vi "DebugMachine Viewer.vi"() -> ()   [LabVIEW 2009]
uses:
  Debug Data Packet.ctl
  TypeDefs/State Machine/Main State.ctl
  cRIO/Functional Global Variables/Status Indicators.ctl
  TypeDefs/Sensor TypeDefs/GPS Data.ctl
  TypeDefs/Sensor TypeDefs/SICK Array.ctl
  Remote Control/Motor Command.ctl
  TypeDefs/Queue TypeDefs/Motor Instruction.ctl
  TypeDefs/Queue TypeDefs/Motor State.ctl
  UDP Lib/UDP Network Location.ctl
  <vilib>/Platform/TimedLoop/XDataNode/XDataNode.xnode
  <vilib>/Platform/TimedLoop/XDataNode/loadlvalarms.vi
  <vilib>/Platform/TimedLoop/XDataNode/timing_clust.ctl
  <vilib>/Platform/TimedLoop/XDataNode/nitl_modes.ctl
  <vilib>/Platform/TimedLoop/XDataNode/wakeup.ctl
  <vilib>/Platform/TimedLoop/XDataNode/XDNodeRunTimeDep.lvlib
panel:
  out "Corrupt Data":bool=TRUE
  in  "Compact RIO Location":T1={"IP Address"="192.168.1.2", "Port"=50004}
  out "Viewer Start time":timestamp=timestamp(3355340375.117 s since 1904-01-01)
  out "Time of most recent data":timestamp=timestamp(3355340545.74 s since 1904-01-01)
  out "Iteration Duration":i64=1000
  out "Timeout":bool=TRUE
  out "HB":bool=TRUE
  in  "stop":bool
  out "Sender Network Location":T1={"IP Address"="0.0.0.0", "Port"=0}
  out "Cluster":T2={"Main State out"=enum."Initialize Sensors", "HB out"=FALSE, "Status Indicators out"={"GPS Init Complete"=FALSE, "SICK Init Complete"=FALSE, "Compass Init Complete"=FALSE, "Camera Init Complete"=FALSE, "Sensors Init Complete"=FALSE, "Motors Init Complete"=FALSE, "MC Heartbeat"=FALSE, "Motors On?"=FALSE}, "RC/!Run out"=TRUE, "AUT/!NAV"=FALSE, "Compass Data"=0.0, "GPS Data"={"Latitude"=0.0, "Longitude"=0.0}, "SICK Data"=[], "Target Bearing"=0.0, "Target Sector"=0, "Calculated sector"=0, "RC Command"={"Speed"=0, "Turn"=0}, "Motor Loop Instruction"={"Motor State"=enum."Stop", "Motor Command"={"Speed"=0, "Turn"=0}}, "Waypoints reached"=0, "Battery Voltage"=0.0} {"GPS Data"."Longitude" format="%#_14g"; "GPS Data"."Latitude" format="%#_14g"}
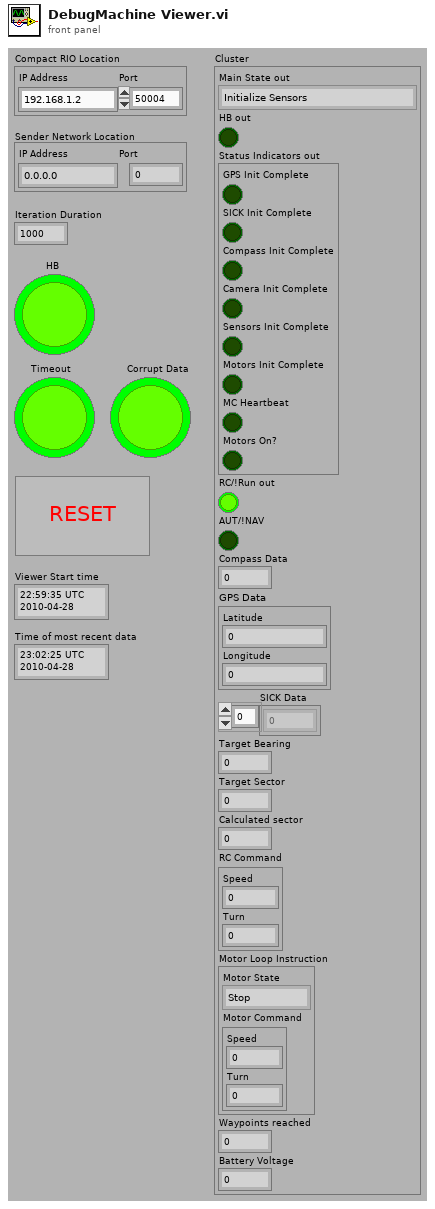
[diagram p1: front panel]
types:
  T1 = typedef "UDP Network Location.ctl" = cluster{"IP Address":string, "Port":u16}
  T2 = typedef "Debug Data Packet.ctl" = cluster{"Main State out":T3, "HB out":bool, "Status Indicators out":T4, "RC/!Run out":bool, "AUT/!NAV":bool, "Compass Data":dbl, "GPS Data":T5, "SICK Data":T6, "Target Bearing":dbl, "Target Sector":i16, "Calculated sector":i16, "RC Command":T7, "Motor Loop Instruction":T8, "Waypoints reached":i8, "Battery Voltage":dbl}
  T3 = typedef "Main State.ctl" = enum16{"Initialize Sensors", "Initialize Motors", "Wait for GO", "Run", "Remote Control", "Stop"}
  T4 = typedef "Status Indicators.ctl" = cluster{"GPS Init Complete":bool, "SICK Init Complete":bool, "Compass Init Complete":bool, "Camera Init Complete":bool, "Sensors Init Complete":bool, "Motors Init Complete":bool, "MC Heartbeat":bool, "Motors On?":bool}
  T5 = typedef "GPS Data.ctl" = cluster{"Latitude":dbl, "Longitude":dbl}
  T6 = typedef "SICK Array.ctl" = u16[]
  T7 = typedef "Motor Command.ctl" = cluster{"Speed":i16, "Turn":i16}
  T8 = typedef "Motor Instruction.ctl" = cluster{"Motor State":T9, "Motor Command":T7}
  T9 = typedef "Motor State.ctl" = enum16{"Wait", "Initialize", "Check FET", "Run", "Stop"}
  T10 = typedef "XDNodeRunTimeDep.lvlib/timing_clust.ctl" = cluster{"Expected End [f-1]":u64, "Actual End [f-1]":u64, "Finished Late? [f-1]":bool, "Expected End [i-1]":u64, "Actual End [i-1]":u64, "Finished Late? [i-1]":bool, "Expected Start [i]":u64, "Actual Start [i]":u64, "Expected Start [f]":u64, "Actual Start [f]":u64, "Source Name":string, "Structure Name":string, "Period":i64, "Deadline":i64, "Offset":i64, "Start":i64, "Priority":i32, "Timeout":i32, "Mode":T11, "Wakeup Reason":T12, "Error":errorcluster, "Source Type":string, "Secondary Source Type":string, "Global End Time":u64, "Global Start Time":u64, "Frame Duration":u64, "Iteration Duration":u64, "Assigned CPU":i32, "I/O Scan Engine Mode":u32}
  T11 = typedef "XDNodeRunTimeDep.lvlib/nitl_modes.ctl" = enum32{"No Change", "Process missed periods, maintain original phase", "Discard missed periods, maintain original phase", "Process missed periods, ignore original phase", "Discard missed periods, ignore original phase"}
  T12 = typedef "XDNodeRunTimeDep.lvlib/wakeup.ctl" = enum32{"Normal", "Aborted", "Asynchronous wakeup", "Timing source error", "Timed loop error", "Timeout"}
  T13 = typedef "UDP Base.ctl" = cluster{"UDP Session":refnum<k16>, "UDP Socket Params":T14}
  T14 = typedef "UDP Socket Params.ctl" = cluster{"Local Port":u16, "Read Timeout":i32, "Write Timeout":i32}
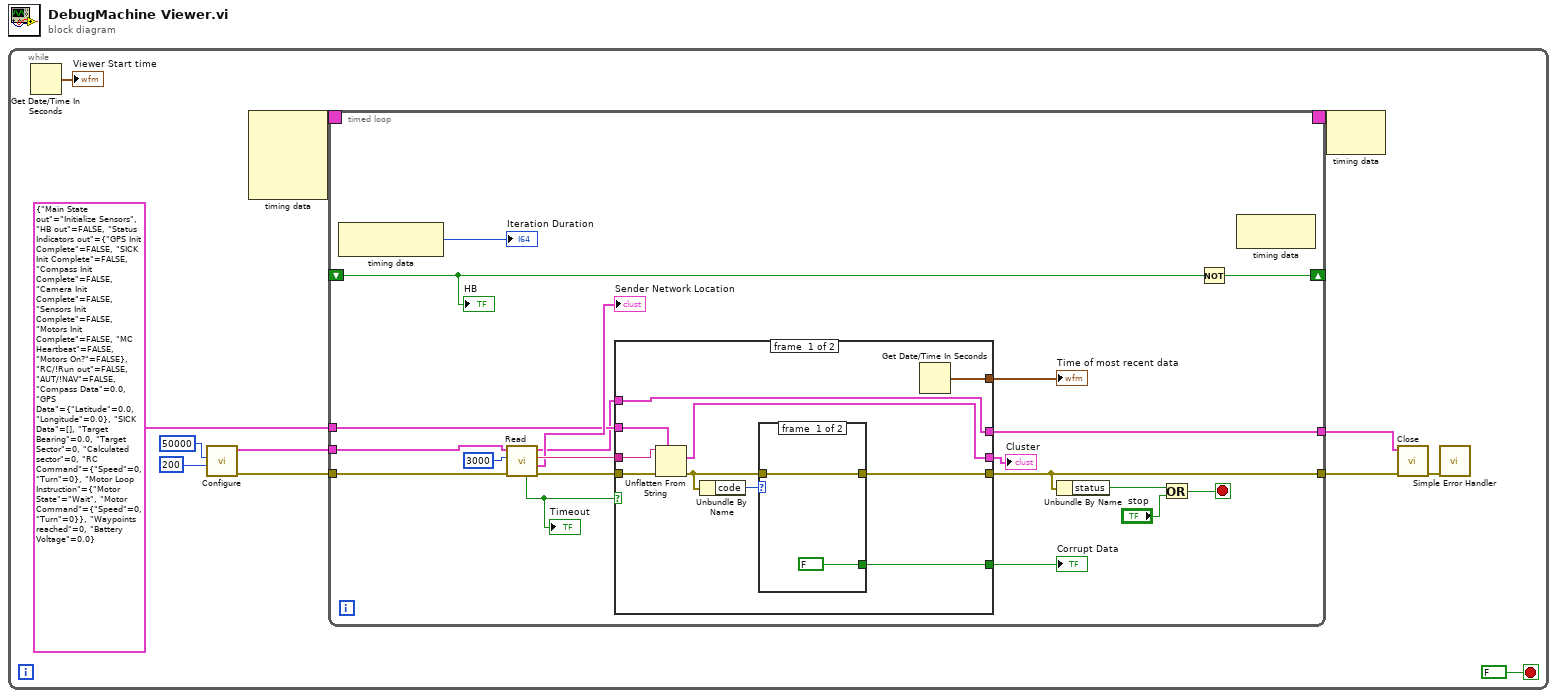
[diagram p0: block diagram]
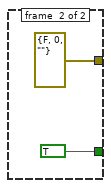
[diagram p2: hidden frame]
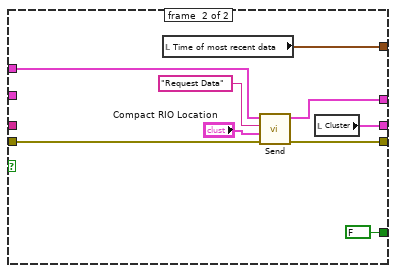
[diagram p3: hidden frame]
diagram:
  n1 = while {
    stop <- FALSE stop-if-true
    n2 = Get Date/Time In Seconds() -> (seconds since 1Jan1904=→"Viewer Start time":timestamp)
    n3 = call "Configure.vi"("Read Timeout"=200, "Local Port"=u16 50000) -> ("error out"=w10:errorcluster, "UDP Base out"=w9:T13)  [unwired: 8 in]
    n4 = node-c288() -> (w12:T10)  [unwired: 4 in]
    n5 = timed-loop {
      timing: w12 -> [_]
      timing-out: [_] -> w11
      tunnel: w10 -> [w31]
      tunnel: w9 -> [w30]
      tunnel: [w24] -> w8
      tunnel: T2 {"Main State out"=enum."Initialize Sensors", "HB out"=FALSE, "Status Indicators out"={"GPS Init Complete"=FALSE, "SICK Init Complete"=FALSE, "Compass Init Complete"=FALSE, "Camera Init Complete"=FALSE, "Sensors Init Complete"=FALSE, "Motors Init Complete"=FALSE, "MC Heartbeat"=FALSE, "Motors On?"=FALSE}, "RC/!Run out"=FALSE, "AUT/!NAV"=FALSE, "Compass Data"=0.0, "GPS Data"={"Latitude"=0.0, "Longitude"=0.0}, "SICK Data"=[], "Target Bearing"=0.0, "Target Sector"=0, "Calculated sector"=0, "RC Command"={"Speed"=0, "Turn"=0}, "Motor Loop Instruction"={"Motor State"=enum."Wait", "Motor Command"={"Speed"=0, "Turn"=0}}, "Waypoints reached"=0, "Battery Voltage"=0.0} ("Cluster") -> [w25]
      shift-right: [w19] -> _
      shift-left: _ -> [w20]
      tunnel: [w15] -> w3
      stop <- w23 stop-if-true
      n6 = node-c288() -> (→"Iteration Duration":i64)  [unwired: 1 in]
      n7 = call "Read.vi"("error in (no error)"=w31, "max size (548)"=3000, "UDP Base in"=w30) -> ("error out"=w29:errorcluster, "Network Location"=→"Sender Network Location":T1, "Receive Data"=w28:string, "UDP Base out"=w16:T13, "Timeout"=w13:bool)  [unwired: 3 in, 1 out]
      "Timeout" <- w13
      n8 = case shown="False" w13 {
        tunnel: w29 -> [w42 w53]
        tunnel: [w33 w50] -> w24
        tunnel: w28 -> [w41 _]
        tunnel: [w40 w55] -> w26
        tunnel: w25 -> [w39 _]
        tunnel: [w38 w54] -> w17
        tunnel: w16 -> [w37 w52]
        tunnel: [w37 w51] -> w15
        tunnel: [w35 FALSE] -> w14
        frame #0 {
          n9 = Unflatten From String(type=w39, binary string=w41, error in (no error)=w42) -> (value=w40:T2, error out=w34:errorcluster)  [unwired: 2 in, 1 out]
          n10 = Unbundle By Name(w34) -> ("code"=w36:i32)
          n11 = case shown="Default" w36 {
            tunnel: [FALSE TRUE] -> w35
            tunnel: w34 -> [w43 _]
            tunnel: [w43 errorcluster {"status"=FALSE, "code"=0, "source"=""} ("error out")] -> w33
            frame #0 {
            }
            frame #1 {
            }
          }
          n12 = Get Date/Time In Seconds() -> (seconds since 1Jan1904=w38:timestamp)
        }
        frame #1 {
          n13 = local read "Time of most recent data"() -> (w54:timestamp)
          n14 = call "Send.vi"("error in (no error)"=w53, "Destination Location"="Compact RIO Location", "Send Data"="Request Data", "UDP Base in"=w52) -> ("error out"=w50:errorcluster, "UDP Base out"=w51:T13)  [unwired: 5 in, 1 out]
          n15 = local read "Cluster"() -> (w55:T2)
        }
      }
      "Cluster" <- w26
      "Time of most recent data" <- w17
      "Corrupt Data" <- w14
      n16 = Unbundle By Name(w24) -> ("status"=w21:bool)
      n17 = Or(x=w21, y="stop") -> (x .or. y?=w23:bool)
      n18 = Not(x=w20) -> (.not. x?=w19:bool)
      n19 = node-c288() -> ()  [unwired: 1 in, 1 out]
      "HB" <- w20
    }
    n20 = node-c288(w11) -> ()  [unwired: 1 out]
    n21 = call "Close.vi"("error in (no error)"=w8, "Cluster of class private data"=w3) -> ("error out"=w2:errorcluster)  [unwired: 9 in]
    n22 = call <vilib>:"Simple Error Handler.vi"("error in (no error)"=w2) -> ()  [unwired: 4 in, 5 out]
  }
